vi "Drop Connection.vi"(8 "error in (no error)":errorcluster, 11 "WebSocket Connection in":refnum<class "WebSocket Connection.lvclass">) -> (0 "error out":errorcluster, 3 "WebSocket Connection out":refnum<class "WebSocket Connection.lvclass">)   [LabVIEW 2021, in "WebSocket Actors.lvlib" / "WebSocket Connection.lvclass"]
doc: "This method drops the connection and is called when the Keepalive Heartbeat times out"
uses:
  WebSocket Connection.lvclass
  C:/Program Files/National Instruments/LabVIEW 2021/vi.lib/ActorFramework/Actor/Actor.lvclass
  Connection Status.ctl
  WebSocket Connection.lvclass/WebSocket Connection.ctl
  <vilib>/ActorFramework/Actor/Actor.lvclass/Actor.ctl
  <vilib>/ActorFramework/Message Enqueuer/Message Enqueuer.lvclass/Message Enqueuer.ctl
  properties/Write Connection Status.vi
  <vilib>/ActorFramework/Message Enqueuer/Init from Existing Queue.vi
  <vilib>/ActorFramework/Message Enqueuer/Enqueue.vi
  <vilib>/ActorFramework/Stop Msg/Stop Msg.lvclass
  C:/Program Files/National Instruments/LabVIEW 2021/vi.lib/ActorFramework/Message/Message.lvclass
  <vilib>/Utility/LVClass/Get LV Class Name.vi
  <resource>/AFDebug/Generate Trace for Message.vi
  <vilib>/ActorFramework/Message Priority Queue/Priority Enqueue.vi
  <vilib>/ActorFramework/Message Enqueuer/Message Enqueuer.lvclass
  <vilib>/ActorFramework/Actor/Actor.lvclass
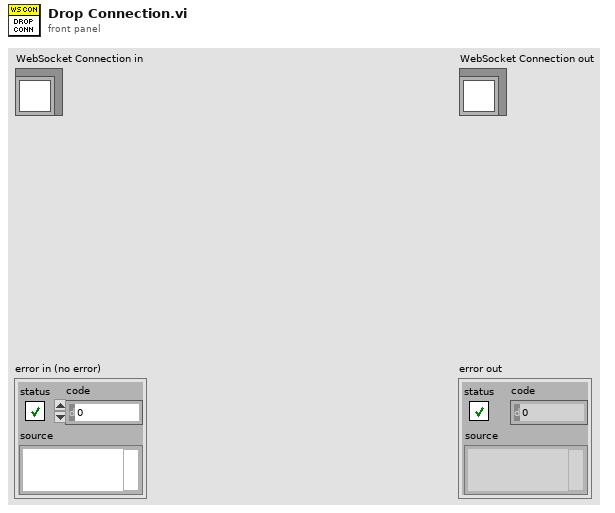
[diagram p1: front panel]
types:
  T1 = typedef "WebSocket Actors.lvlib/WebSocket Connection.lvclass/Connection Status.ctl" = enum16{"Open", "Closed by Self", "Closed by Peer", "Dropped"}
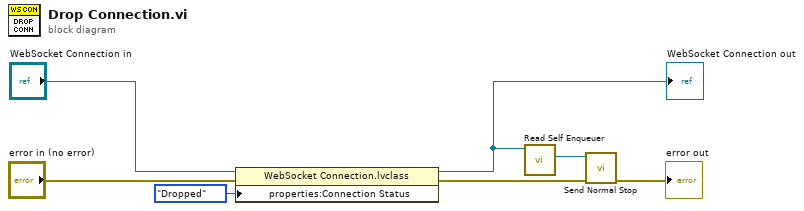
[diagram p0: block diagram]
diagram:
  n1 = property class="WebSocket Connection.lvclass"(reference="WebSocket Connection in", error in="error in (no error)", "properties:Connection Status"=Connection_Status."Dropped" ("Connection Status")) -> (reference out=w2:refnum<class "WebSocket Connection.lvclass">, error out=w3:errorcluster)
  "WebSocket Connection out" <- w2
  n2 = call <vilib>:"Read Self Enqueuer.vi"("Actor"=w2) -> ("Self Enqueuer"=w1:refnum<class "Message Enqueuer.lvclass">)  [unwired: 10 in]
  n3 = call <vilib>:"Send Normal Stop.vi"("error in (no error)"=w3, "Message Enqueuer"=w1) -> ("error out"=→"error out":errorcluster)  [unwired: 9 in]
